vi "SaveDialog.vi"(8 "error in":errorcluster, 11 "state in":T1) -> (0 "error out":errorcluster, 1 "new":bool, 3 "state out":T1)   [LabVIEW 2013, in "vi mod UI.lvlib"]
uses:
  vi mod UI.lvlib
  Controls/StateCluster.ctl
  <vilib>/NI/Configuration Framework/Repository/NISE_CEF_Repository.lvclass
  <vilib>/NI/Configuration Framework/Node/NodeRef.ctl
  <vilib>/NI/Configuration Framework/Node/NISE_CEF_Node.lvclass
  <vilib>/NI/Configuration Framework/Node/UserEventRef.ctl
  <vilib>/NI/Configuration Framework/Controls/EventCluster.ctl
  <vilib>/NI/Configuration Framework/NISE_CEF_TreeControl.lvlib
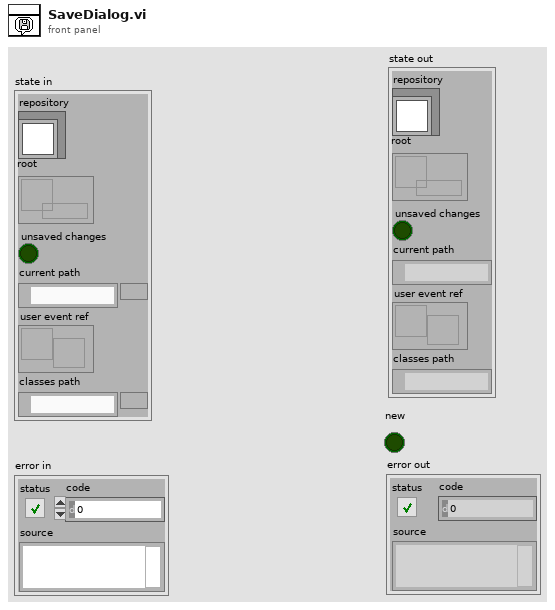
[diagram p1: front panel]
types:
  T1 = typedef "vi mod UI.lvlib/StateCluster.ctl" = cluster{"repository":refnum<class "NISE_CEF_Repository.lvclass">, "root":T2, "unsaved changes":bool, "current path":path, "user event ref":T3, "classes path":path}
  T2 = typedef "NISE_CEF_Node.lvclass/NodeRef.ctl" = refnum<data-value>
  T3 = typedef "NISE_CEF_Node.lvclass/UserEventRef.ctl" = refnum<user-event>
  T4 = enum16{"Left Button", "Center Button", "Right Button", "Window Close"}
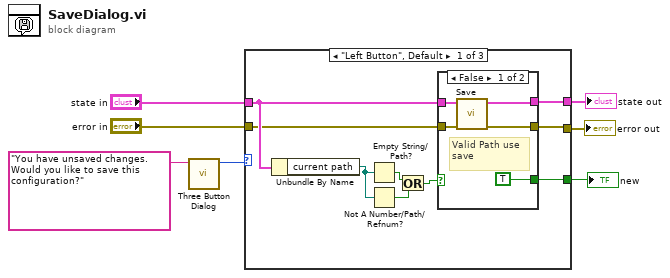
[diagram p0: block diagram]
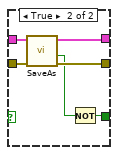
[diagram p2: hidden frame]
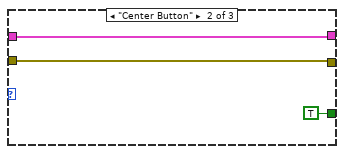
[diagram p3: hidden frame]
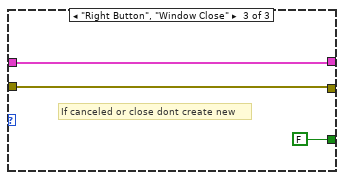
[diagram p4: hidden frame]
diagram:
  n1 = call <vilib>:"Three Button Dialog.vi"("message"="You have unsaved changes.  Would you like to save this configuration?") -> ("Which Button?"=w2:T4)  [unwired: 10 in]
  n2 = case shown="\"Left Button\", Default" w2 {
    tunnel: "state in" -> [w12 w29 w32]
    tunnel: [w11 w29 w32] -> w6
    tunnel: "error in" -> [w9 w28 w31]
    tunnel: [w10 w28 w31] -> w4
    tunnel: [w8 TRUE ("New") FALSE ("New")] -> w1
    frame "Left Button", Default {
      n3 = Unbundle By Name(w12) -> ("current path"=w16:path)
      n4 = Empty String/Path?(string/path=w16) -> (empty?=w14:bool)
      n5 = Not A Number/Path/Refnum?(number/path/refnum=w16) -> (NaN/Path/Refnum?=w13:bool)
      n6 = Or(x=w14, y=w13) -> (x .or. y?=w15:bool)
      n7 = case shown="False" w15 {
        tunnel: w12 -> [w21 w25]
        tunnel: [w20 w24] -> w11
        tunnel: [w19 w26] -> w10
        tunnel: w9 -> [w18 w27]
        tunnel: [TRUE w22] -> w8
        frame False {
          # "Valid Path use save"
          n8 = call "Save.vi"("error in"=w18, "state in"=w21) -> ("error out"=w19:errorcluster, "state out"=w20:T1)  [unwired: 8 in]
        }
        frame True {
          n9 = call "SaveAs.vi"("error in"=w27, "state in"=w25) -> ("error out"=w26:errorcluster, "canceled?"=w23:bool, "state out"=w24:T1)  [unwired: 7 in]
          n10 = Not(x=w23) -> (.not. x?=w22:bool)
        }
      }
    }
    frame "Center Button" {
    }
    frame "Right Button", "Window Close" {
      # "If canceled or close dont create new"
    }
  }
  "state out" <- w6
  "error out" <- w4
  "new" <- w1
